vi "Rinse System.vi"(8 "error in (no error)":errorcluster) -> (0 "error out":errorcluster)   [LabVIEW 2018, in "cetoni.lvlib" / "cetoni.lvclass"]
uses:
  cetoni.lvclass
  <userlib>/QmixLib/QmixLib.lvlib
  Program Files/cetoni/QmixSDK/lib/labview/labbCAN_Pump_API/labbCAN_Pump_API.lvlib
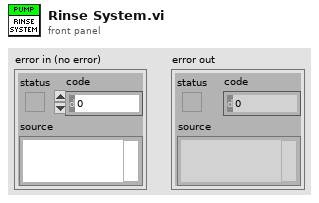
[diagram p1: front panel]
types:
  T1 = enum16{"Left Button", "Center Button", "Right Button", "Window Close"}
  T2 = enum16{"LOW_PRESSURE_VALVE", "BALL_VALVE", "QMIX_VALVE"}
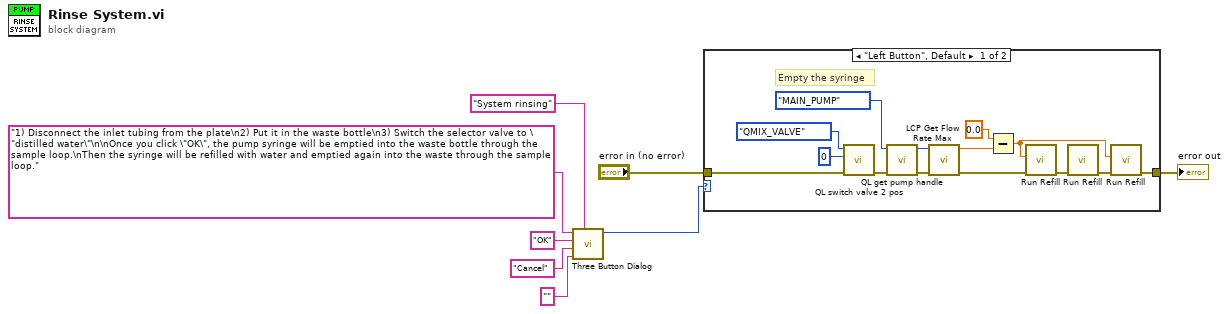
[diagram p0: block diagram]
diagram:
  n1 = call <vilib>:"Three Button Dialog.vi"("Window Title (\"\")"="System rinsing" ("Window Title (\"\")"), "Right Button Text (\"Cancel\")"="" ("Right Button Text (\"Cancel\")"), "Center Button Text (\"No\")"="Cancel" ("Center Button Text (\"No\")"), "Left Button Text (\"Yes\")"="OK" ("Left Button Text (\"Yes\")"), "message"="1) Disconnect the inlet tubing from the plate\n2) Put it in the waste bottle\n3) Switch the selector valve to \"distilled water\"\n\nOnce you click \"OK\", the pump syringe will be emptied into the waste bottle through the sample loop.\nThen the syringe will be refilled with water and emptied again into the waste through the sample loop.") -> ("Which Button?"=w3:T1)  [unwired: 6 in]
  n2 = case shown="\"Left Button\", Default" w3 {
    tunnel: [w17 w23] -> w2
    tunnel: "error in (no error)" -> [w21 w23]
    frame "Left Button", Default {
      # "Empty the syringe"
      n3 = call <userlib>:"QL switch valve 2 pos.vi"("error in (no error)"=w21, "pos"=0, "valve"=T2."QMIX_VALVE") -> ("error out"=w16:errorcluster)  [unwired: 8 in]
      n4 = call <userlib>:"QL get pump handle.vi"("error in (no error)"=w16, "pump"=enum16{"MAIN_PUMP"}."MAIN_PUMP") -> ("error out"=w15:errorcluster, "pump handle"=w14:u64)  [unwired: 8 in]
      n5 = call "LCP Get Flow Rate Max.vi"("error in (no error)"=w15, "Pump Handle"=w14) -> ("error out"=w10:errorcluster, "Maximum Flow Rate"=w11:dbl)  [unwired: 8 in]
      n6 = Subtract(x=0.0, y=w11) -> (x-y=w9:dbl)
      n7 = call "Run Refill.vi"("error in (no error)"=w10, "flow_rate_uL_s"=w9) -> ("error out"=w19:errorcluster)  [unwired: 9 in]
      n8 = call "Run Refill.vi"("error in (no error)"=w19) -> ("error out"=w18:errorcluster)  [unwired: 10 in]
      n9 = call "Run Refill.vi"("error in (no error)"=w18, "flow_rate_uL_s"=w9) -> ("error out"=w17:errorcluster)  [unwired: 9 in]
    }
    frame "Center Button" {
    }
  }
  "error out" <- w2
